vi "CAN Statuswerte.vi"() -> (2 "CAN data":T1[](array[typedef])=[{"timestamp"=timestamp(0 s since 1904-01-01), "payload"=[0, 2, 3, 4, 5, 6, 7, 8], "identifier"=2, "type"=0, "extended?"=FALSE, "echo?"=FALSE}, {"timestamp"=timestamp(0 s since 1904-01-01), "payload"=[0, 1, 2, 3, 4, 5, 6, 7], "identifier"=3, "type"=0, "extended?"=FALSE, "echo?"=FALSE}] {"payload" format="%x"; "timestamp" format="%<%.7X\n%x>T"; "type" items=["CAN Data"=0, "CAN Remote"=1, "CAN Bus Error"=2, "CAN 2.0 Data"=8, "CAN FD Data"=16, "CAN FD+BRS Data"=24, "J1939 Data"=192, "Delay"=224, "Log Trigger"=225, "Start Trigger"=226]; "identifier" format="%x"})   [LabVIEW 2020]
uses:
  195161_2023-03-15/cRIO/CAN Interface/CAN Interface.lvlib
  FGV CAN Daten Aktionen.ctl
  195161_2023-03-15/cRIO/Verwaltung/Verwaltung - cRIO.lvlib
  Verwaltung/FGV IN Aktionen.ctl
  195161_2023-03-15/cRIO/Stoermeldungen/Stoermeldungen.lvlib
  Stoermeldungen/FGV Stoerungen Aktionen.ctl
  Axetris-Laser/Kalibrierung/Aktion FGV Messwerte.ctl
  195161_2023-03-15/cRIO/Allgemein/Allgemein.lvlib
  Allgemein/FGV Zustaende Aktionen.ctl
  Allgemein/FGV Spuelung Aktionen.ctl
  Allgemein/Zustaende.ctl
  <vilib>/xnet/xnet.llb/XNET Frame Type CAN.ctl
  <vilib>/xnet/xnet.llb/XNET Frame CAN.ctl
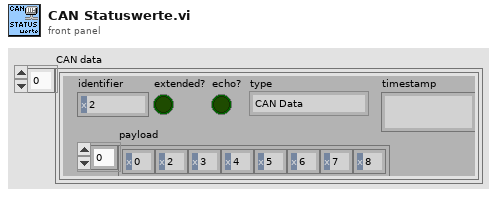
[diagram p1: front panel]
types:
  T1 = typedef "XNET Frame CAN.ctl" = cluster{"timestamp":timestamp, "payload":u8[], "identifier":u32, "type":T2, "extended?":bool, "echo?":bool}
  T2 = typedef "XNET Frame Type CAN.ctl" = u8
  T3 = typedef "Allgemein.lvlib/Zustaende.ctl" = enum16{"PAUSE", "Standby", "Messen", "Kalibrieren 0", "Kalibrieren E", "Spülen Filter", "Spülen Leitung", "CalGas", "0-Gas", "Hintergrund", "Linearisierung"}
  T4 = typedef "Allgemein.lvlib/FGV Spuelung Aktionen.ctl" = enum16{"lesen", "Spülen", "Testmodus", "Kal.zustand rücksetzen", "initialisieren", "Aufzeichnung"}
  T5 = typedef "Allgemein.lvlib/FGV Zustaende Aktionen.ctl" = enum16{"lesen", "Zustand PC", "Zustand cRIO", "Bildnummer", "Samplepoint", "Sysloglevel"}
  T6 = typedef "Axetris-Laser.lvlib/Kalibrierung.lvlib/Aktion FGV Messwerte.ctl" = enum16{"lesen", "CAL-Daten laden", "Messen", "Kalibrieren vorbereiten", "Kalibrieren", "CAL-Daten speichern", "Toleranz schreiben", "CAL-Daten kopieren", "Polynom", "LIN aktiv", "Polynom Daten speichern", "Rohwert vor Lin", "Rohwert nach Lin", "RefDruck setzen"}
  T7 = typedef "Stoermeldungen.lvlib/FGV Stoerungen Aktionen.ctl" = enum16{"lesen", "Störung aktiv?", "1-64", "65-128"}
  T8 = typedef "Verwaltung - cRIO.lvlib/FGV IN Aktionen.ctl" = enum16{"lesen", "DI", "AI", "Fühler Br.", "TC", "Fühler Br. TC"}
  T9 = typedef "CAN Interface.lvlib/FGV CAN Daten Aktionen.ctl" = enum16{"lesen", "Daten", "Konfig", "laden", "speichern", "Status"}
  T10 = typedef "Verwaltung - cRIO.lvlib/Analog Eingaenge.ctl" = cluster{"AI0: Durchfluss":sgl, "AI1: Druck Messzelle":sgl, "AI2: Druck Umgebung":sgl, "AI3: Batterieanzeige":sgl, "AI4: Reserve":sgl, "AI5: Reserve":sgl, "AI6: Trigger":sgl, "AI7: Reserve":sgl, "Rohwert Durchfluss LGD":sgl, "Rohwert Druck Messzelle":sgl, "Rohwert Druck Umgebung":sgl, "TC0: Temp. Aussen":sgl, "TC1: HL":sgl, "TC2: Filter":sgl, "TC3: Temp. Bereich LGD":sgl, "TC4: Reserve":sgl, "TC5: Reserve":sgl, "TC6: Reserve":sgl, "TC7: Reserve":sgl, "TC8: Reserve":sgl, "TC9: Reserve":sgl, "TC10: Reserve":sgl, "TC11: Reserve":sgl, "TC12: Reserve":sgl, "TC13: Reserve":sgl, "TC14: Reserve":sgl, "TC15: Reserve":sgl}
  T11 = typedef "CAN Konfig.lvlib/Konfig Daten PC.ctl" = cluster{"Baude Rate":T12, "COM state":u8, "Frame-ID FTIR Start":u32, "Frame-ID FTIR End":u32, "Frame-ID Status Start":u32, "Frame-ID Status End":u32, "Zustand Information":u32, "Aktion":u32, "Frame-ID FTIR Arry":u32[], "Frame-ID Status Arry":u32[], "GPS Start":u32, "Interface":refnum<k21>}
  T12 = typedef "CAN Interface.lvlib/Baude Rate.ctl" = u32
  T13 = typedef "Funktionstasten.lvlib/Zustaende.ctl" = enum16{"Standby", "Pause", "Eco", "Messen", "Kalibrieren", "Spülen Filter", "Spülen Leitung", "Umgebungsluft", "0-Gas", "Cal-Gas", "CG zu PNS", "-------------", "Init 1", "Init 2", "Init 3", "Init 4", "Messen vorbereiten", "Messen durchführen", "Exit"}
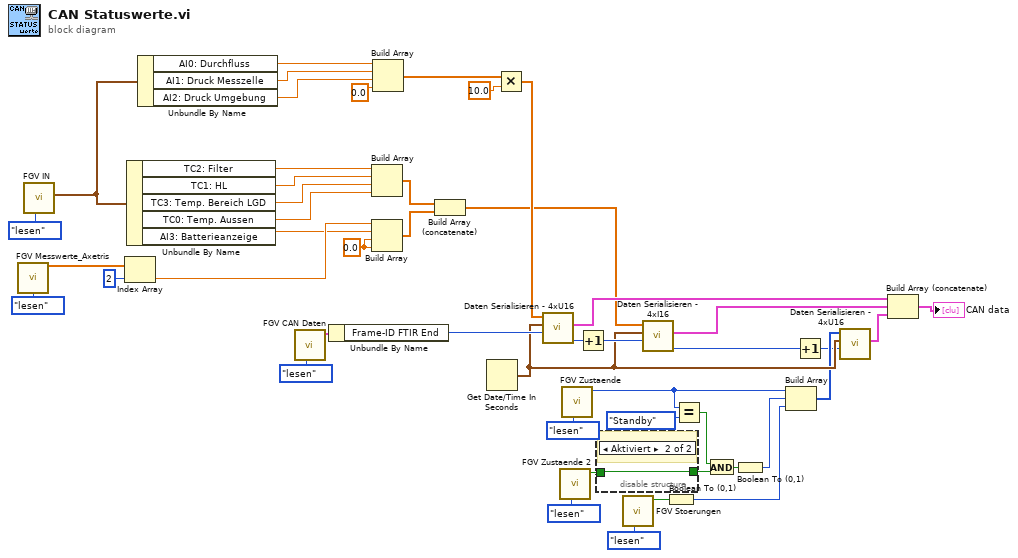
[diagram p0: block diagram]
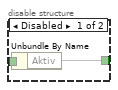
[diagram p2: hidden frame]
diagram:
  w21 = sgl 0.0 ("Element")
  n1 = call "FGV Messwerte_Axetris.vi"("Aktion"=Aktion_FGV_Messwerte."lesen") -> ("GasValue"=w24:sgl[])  [unwired: 9 in, 5 out]
  n2 = call "FGV IN.vi"("Aktion"=FGV_IN_Aktionen."lesen") -> ("Analog Eingänge"=w35:T10)  [unwired: 8 in, 2 out]
  n3 = Index Array(array=w24, index=2 ("Index")) -> (element=w22:sgl)
  n4 = Unbundle By Name(w35) -> ("TC2: Filter"=w34:sgl, "TC1: HL"=w33:sgl, "TC3: Temp. Bereich LGD"=w32:sgl, "TC0: Temp. Aussen"=w31:sgl, "AI3: Batterieanzeige"=w1:sgl)
  n5 = Unbundle By Name(w35) -> ("AI0: Durchfluss"=w44:sgl, "AI1: Druck Messzelle"=w43:sgl, "AI2: Druck Umgebung"=w36:sgl)
  n6 = call "FGV CAN Daten.vi"("Aktionen"=FGV_CAN_Daten_Aktionen."lesen") -> ("Konfig Daten"=w47:T11)  [unwired: 8 in, 2 out]
  n7 = Unbundle By Name(w47) -> ("Frame-ID FTIR End"=w45:u32)
  n8 = Build Array(w34, w33, w32, w31) -> (w20:sgl[])
  n9 = Build Array(w22, w1, w21, w21) -> (w19:sgl[])
  n10 = Build Array(w44, w43, w36, sgl 0.0 ("Element")) -> (w27:sgl[])
  n11 = Build Array (concatenate)(w20, w19) -> (w18:sgl[])
  n12 = Get Date/Time In Seconds() -> (seconds since 1Jan1904=w17:timestamp)
  n13 = Multiply(x=w27, y=sgl 10.0) -> (x*y=w28:sgl[])
  n14 = call "Daten Serialisieren - 4xU16.vi"("Frame-ID"=w45, "Aktuelle Zeit"=w17, "Messdaten"=w28) -> ("Frame-ID letzter Wert"=w42:u32, "data"=w41:T1[])  [unwired: 7 in]
  n15 = call "FGV Zustaende 2.vi"("Aktion"=FGV_Spuelung_Aktionen."lesen") -> ("Spülen"=w16:bool)  [unwired: 8 in, 2 out]
  n16 = call "FGV Zustaende.vi"("Aktionen"=FGV_Zustaende_Aktionen."lesen") -> ("Zustand PC"=w5:T13)  [unwired: 6 in, 4 out]
  n17 = Increment(x=w42) -> (x+1=w39:u32)
  n18 = disable-structure shown="Aktiviert" {
    disable-tunnel: w16 -> [w49 w50]
    disable-tunnel: [w48 w50] -> w2
    frame Disabled {
      n19 = Unbundle By Name(w49) -> ("Aktiv"=w48)
    }
    frame Enabled {
      # "#CanBus"
    }
  }
  n20 = call "FGV Stoerungen.vi"("Aktionen"=FGV_Stoerungen_Aktionen."lesen") -> ("Störung aktiv?"=w8:bool)  [unwired: 8 in, 2 out]
  n21 = call "Daten Serialisieren - 4xI16.vi"("Frame-ID"=w39, "Aktuelle Zeit"=w17, "Messdaten"=w18) -> ("Frame-ID letzter Wert"=w9:u32, "data"=w38:T1[])  [unwired: 7 in]
  n22 = Boolean To (0,1)(Boolean=w8) -> (0, 1=w7:i16)
  n23 = Equal?(x=w5, y=Zustaende."Standby") -> (x = y?=w3:bool)
  n24 = And(x=w3, y=w2) -> (x .and. y?=w6:bool)
  n25 = Boolean To (0,1)(Boolean=w6) -> (0, 1=w15:i16)
  n26 = Build Array(w5, w15, w7) -> (w12:u16[])
  n27 = Increment(x=w9) -> (x+1=w10:u32)
  n28 = call "Daten Serialisieren - 4xU16.vi"("Frame-ID"=w10, "Aktuelle Zeit"=w17, "Messdaten"=w12) -> ("data"=w11:T1[])  [unwired: 7 in, 1 out]
  n29 = Build Array (concatenate)(w41, w38, w11) -> (→"CAN data":T1[])
